vi "Example1.2-8PSK Simulation.vi"() -> ()   [LabVIEW 2013]
uses:
  <vilib>/addons/Modulation/Digital/General/MT Generate Bits (Galois, PN Order).vi
  <vilib>/addons/Modulation/Digital/General/MT Generate PSK System Parameters(M).vi
  <vilib>/addons/Modulation/Digital/General/MT Generate PSK Synchronization Parameters (bit array).vi
  <vilib>/addons/Modulation/Digital/General/MT Format Eye Diagram (complex).vi
  <vilib>/addons/Modulation/niDMT.lvlib
panel:
  out "sync found index (symbols)":dbl format="%.4f"
  in  "Eb/N0 (dB)":dbl(slide)=48.26086956521739 scale=-10.0..50.0
  out "measurements":T1 caption="Measurements" {"phase offset (deg)" format="%.2f"; "frequency drift (Hz)" format="%.2f"; "frequency offset (Hz)" format="%.2f"}
  out "Baseband Waveform":cluster{"t0":dbl, "dt":dbl, "Y":dbl[]}(graph)={"t0"=0.0, "dt"=0.0625, "Y"=array[5376 elements]}
  in  "Tab Control":enum32{"Constellation", "Eye Diagram"}(tab)
  out "Constellation Plot":T2(graph)
  out "Eye Diagram":cluster{"t0":dbl, "dt":dbl, "Y":dbl[]}[](graph)
  in  "M-PSK (4)":i32=8
  out "LED Array":T3
  in  "Message Bits":i32=1000
  in  "stop 2":bool
  out "error out":errorcluster
  # "8-PSK Simulation"
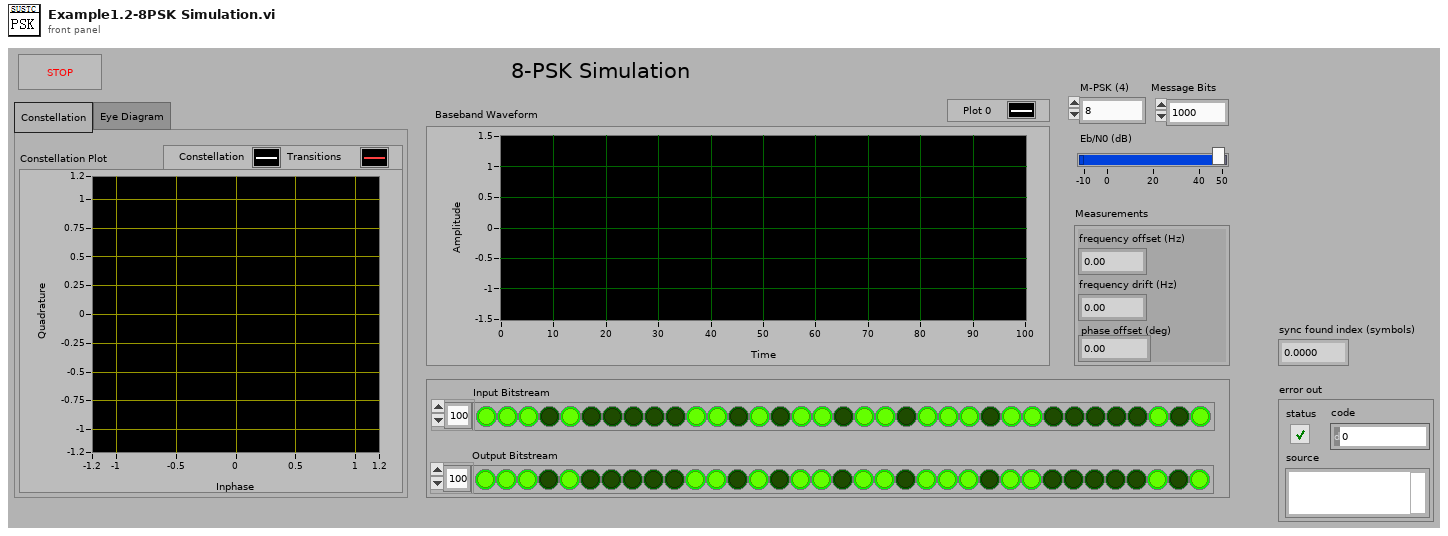
[diagram p1: front panel]
types:
  T1 = cluster{"frequency offset (Hz)":dbl, "frequency drift (Hz)":dbl, "phase offset (deg)":dbl}
  T2 = cluster{"constellation":dbl[], "oversampled data":dbl[]}[]
  T3 = cluster{"Input Bitstream":bool[], "Output Bitstream":bool[]}
  T4 = enum16{"none", "Raised Cosine", "Root Raised Cos", "Gaussian"}
  T5 = enum16{"FSK", "PSK", "QAM", "MSK", "PAM", "ASK", "CPM"}
  T6 = cluster{"samples per symbol (16)":i32, "symbol map":cdb[], "differential PSK":enum16{"disable", "enable"}, "PSK type":u16}
  T7 = typedef "niAMT.lvlib/Complex Data Waveform.ctl" = cluster{"t0":dbl, "dt":dbl, "Y":cdb[]}
  T8 = cluster{"expected sync location (symbols)":i32, "sync sequence":cdb[], "sync location uncertainty (symbols)":i32, "sync indent (symbols)":i32}
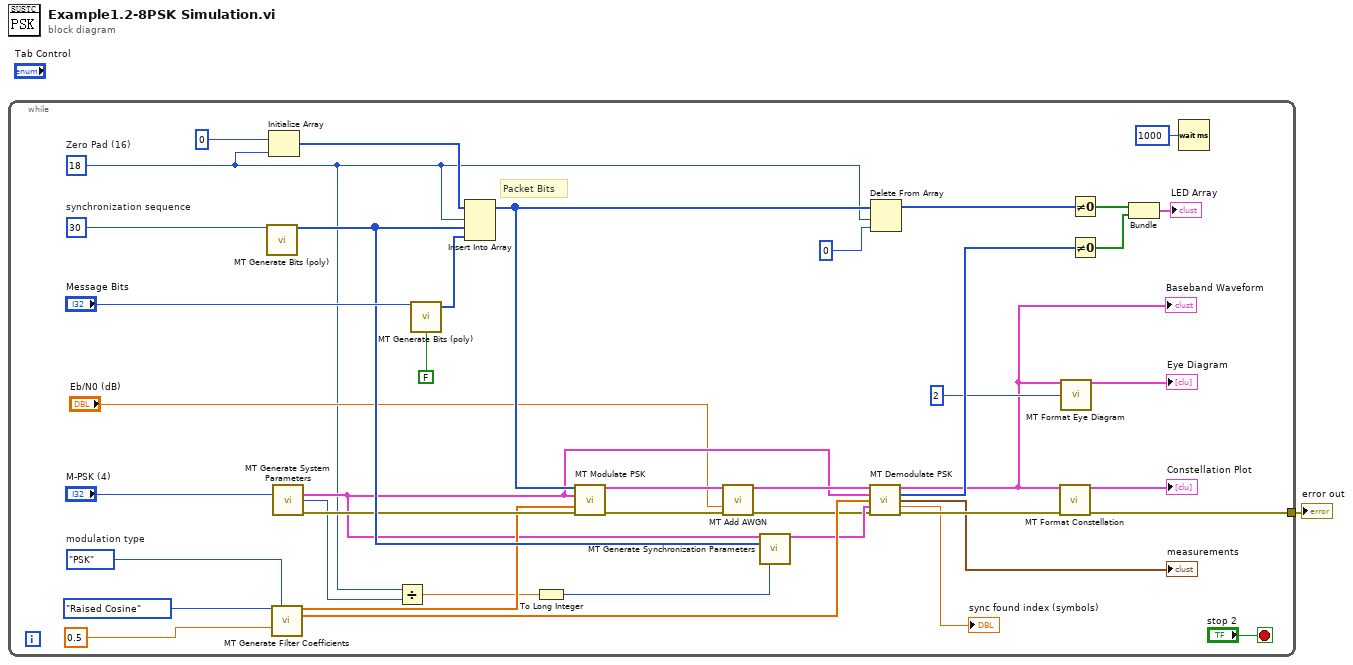
[diagram p0: block diagram]
diagram:
  n1 = while {
    tunnel: [w22] -> w1
    stop <- "stop 2" stop-if-true
    w4 = 18  # Zero Pad (16)
    w34 = 30  # synchronization sequence
    w43 = T5."PSK"  # modulation type
    # "Packet Bits"
    n2 = call-poly <vilib>:"MT Generate Bits (poly).vi"("total bits (128)"=w34) -> ("output bit stream"=w29:i8[])  [unwired: 12 in, 2 out]
    n3 = Initialize Array(i8 0 ("element"), w4) -> (w26:i8[])
    n4 = call <vilib>:"MT Generate Filter Coefficients.vi"("pulse shaping filter (none)"=T4."Raised Cosine", "modulation type"=w43, "filter parameter"=0.5) -> ("pulse shaping filter coefficients"=w14:dbl[], "matched filter coefficients"=w35:dbl[])  [unwired: 10 in, 1 out]
    n5 = call-poly <vilib>:"MT Generate System Parameters.vi"("M-PSK (4)"="M-PSK (4)") -> ("PSK system parameters"=w10:T6, "bits per symbol"=w5:i32, "error out"=w24:errorcluster)  [unwired: 12 in]
    n6 = Divide(x=w4, y=w5) -> (x/y=w3:dbl)
    n7 = call-poly <vilib>:"MT Generate Bits (poly).vi"("total bits (128)"="Message Bits", "reset? (T)"=FALSE) -> ("output bit stream"=w30:i8[])  [unwired: 11 in, 2 out]
    n8 = Insert Into Array(array=w26, index=w4, new element #1=w29, new element #2=w30) -> (w33:i8[])
    n9 = To Long Integer(number=w3) -> (32bit integer=w2:i32)
    n10 = call <vilib>:"MT Modulate PSK.vi"("input bit stream"=w33, "PSK system parameters"=w10, "pulse shaping filter coefficients"=w14, "error in (no error)"=w24) -> ("output complex waveform"=w13:T7, "error out"=w8:errorcluster)  [unwired: 9 in, 1 out]
    n11 = call <vilib>:"MT Add AWGN.vi"("input complex waveform"=w13, "Eb/N0 (10 dB)"="Eb/N0 (dB)", "error in (no error)"=w8) -> ("output complex waveform"=w12:T7, "error out"=w9:errorcluster)  [unwired: 10 in, 1 out]
    n12 = call-poly <vilib>:"MT Generate Synchronization Parameters.vi"("PSK system parameters"=w10, "sync bits"=w29, "expected sync location (symbols)"=w2) -> ("PSK synchronization parameters"=w28:T8)  [unwired: 11 in, 1 out]
    n13 = call <vilib>:"MT Demodulate PSK.vi"("input complex waveform"=w12, "PSK system parameters"=w10, "matched filter coefficients"=w35, "synchronization parameters"=w28, "error in (no error)"=w9) -> ("recovered complex waveform"=w18:T7, "output bit stream"=w38:i8[], "measurements"=→"measurements":T1, "sync found index (symbols)"=→"sync found index (symbols)":dbl, "error out"=w23:errorcluster)  [unwired: 6 in]
    "Baseband Waveform" <- w18
    n14 = Delete From Array(array=w33, length=w4, index=0) -> (array with subset deleted=w31:i8[])  [unwired: 1 out]
    n15 = call <vilib>:"MT Format Constellation.vi"("waveform"=w18, "error in (no error)"=w23) -> ("constellation graph"=→"Constellation Plot":T2, "error out"=w22:errorcluster)  [unwired: 12 in]
    n16 = call-poly <vilib>:"MT Format Eye Diagram.vi"("waveform"=w18, "eye length"=2) -> ("eye diagram"=→"Eye Diagram":cluster{"t0":dbl, "dt":dbl, "Y":dbl[]}[])  [unwired: 12 in, 1 out]
    n17 = Not Equal To 0?(x=w31) -> (x != 0?=w41:bool[])
    n18 = Not Equal To 0?(x=w38) -> (x != 0?=w40:bool[])
    n19 = Bundle(w41, w40) -> (→"LED Array":cluster{bool[], bool[]})  [unwired: 1 in]
    n20 = Wait (ms)(milliseconds to wait=u32 1000) -> ()  [unwired: 1 out]
  }
  "error out" <- w1
